vi "TagBus_Write data dictionary.vi"(10 "tag bus:data dictionary":refnum<class "data dictionary.lvclass">, 11 "TagBus in":refnum<class "TagBus.lvclass">) -> (3 "TagBus out":refnum<class "TagBus.lvclass">)   [LabVIEW 2015, in "TagBus.lvclass"]
uses:
  TagBus.lvclass
  <vilib>/NI/Tag Bus/dictionary/data dictionary.lvclass
  TagBus.lvclass/TagBus.ctl
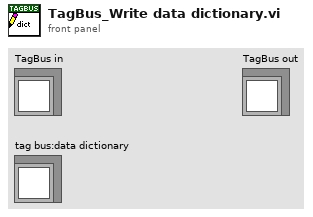
[diagram p1: front panel]
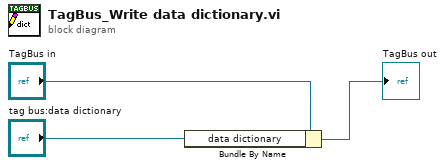
[diagram p0: block diagram]
diagram:
  n1 = Bundle By Name(cluster="TagBus in", "data dictionary"="tag bus:data dictionary") -> (→"TagBus out":refnum<class "TagBus.lvclass">)
